vi "verify parameters in a list.vi"(8 "error in (no error)":errorcluster, 11 "Simulated_CCD_Camera in":refnum<class "Sim_Ixon_Ultra.lvclass">) -> (0 "error out":errorcluster, 3 "Simulated_CCD_Camera out":refnum<class "Sim_Ixon_Ultra.lvclass">)   [LabVIEW 2018, in "Sim_Ixon_Ultra.lvclass"]
doc: "Verify if the parameters of the camera are in range\n\nThe operating parameters of the CCDs must be within a predefined range. This function verifies if the values provided for these parameters meet this specification. If not, ACS will not allow to start an exposure."
uses:
  Sim_Ixon_Ultra.lvclass
  C:/Users/Denis/Desktop/S4ACS/S4ACS/Simulated_CCD_Camera/Simulated Camera.lvclass
  Simulated_CCD_Camera/Simulated Camera.lvclass
panel:
  out "New CCD Config":T1
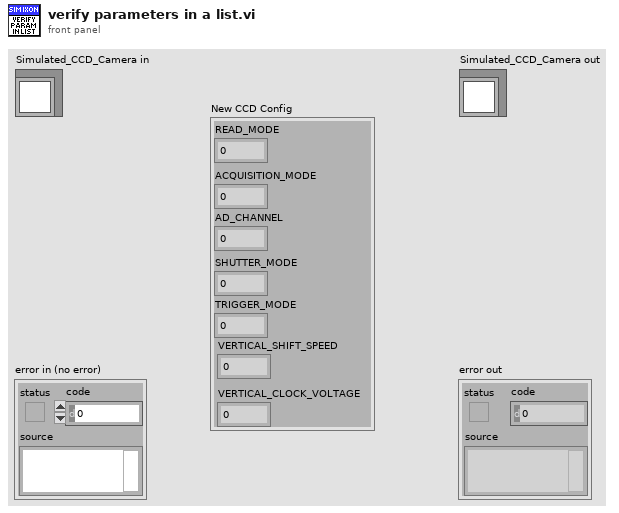
[diagram p1: front panel]
types:
  T1 = cluster{"READ_MODE":u16, "ACQUISITION_MODE":u16, "AD_CHANNEL":u16, "SHUTTER_MODE":u16, "TRIGGER_MODE":u16, "VERTICAL_SHIFT_SPEED":u16, "VERTICAL_CLOCK_VOLTAGE":u16}
  T2 = cluster{"PREAMP":u16, "READOUT_RATE":u16, "VERTICAL_SHIFT_SPEED":u16, "READ_MODE":u16, "VERTICAL_CLOCK_VOLTAGE":u16, "ACQUISITION_MODE":u16, "AD_CHANNEL":u16, "SHUTTER_TTL":u16, "SHUTTER_OPENING_TIME":u16, "SHUTTER_CLOSING_TIME":u16, "SHUTTER_MODE":u16, "TRIGGER_MODE":u16, "VBIN":u16, "INITIAL_LINE":u16, "INITIAL_COLUMN":u16, "FINAL_LINE":u16, "FINAL_COLUMN":u16, "HBIN":u16, "TEMP":u16, "COOLER_POWER_STATUS":u16}
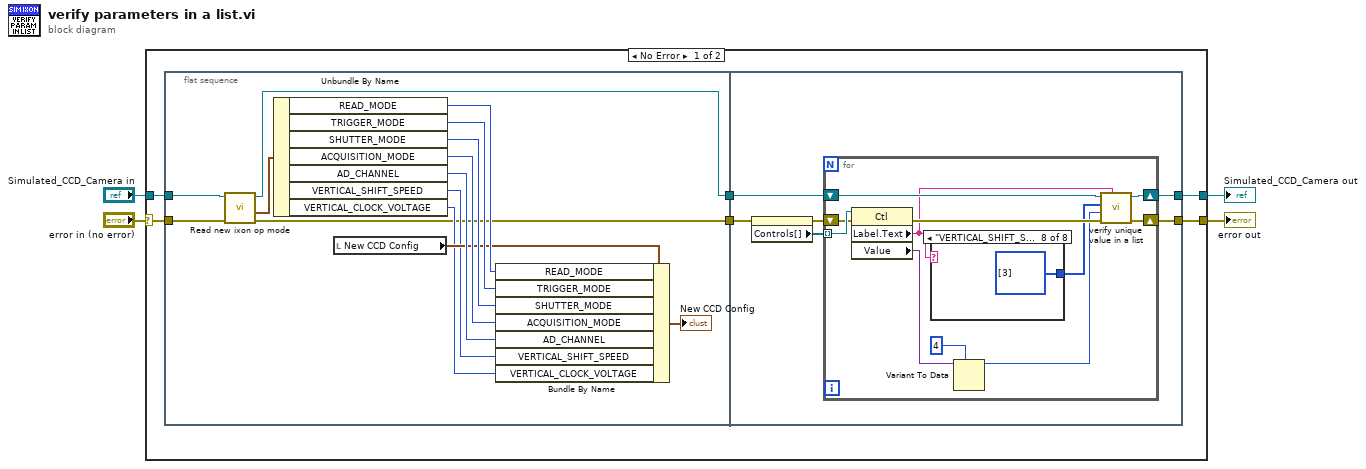
[diagram p0: block diagram]
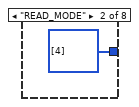
[diagram p3: hidden frame]
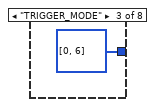
[diagram p4: hidden frame]
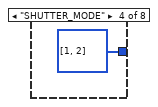
[diagram p5: hidden frame]
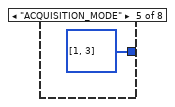
[diagram p6: hidden frame]
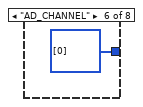
[diagram p7: hidden frame]
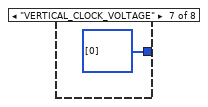
[diagram p8: hidden frame]
diagram:
  n1 = case shown="No Error" "error in (no error)" {
    selector: "error in (no error)" -> [w8 w49]
    tunnel: "Simulated_CCD_Camera in" -> [w7 w50]
    tunnel: [w6 w50] -> w2
    tunnel: [w5 w49] -> w1
    frame No Error {
      n2 = flat-sequence {
        tunnel: w8 -> [w13]
        tunnel: w7 -> [w14]
        tunnel: [w11] -> w10
        tunnel: [w12] -> w9
        tunnel: [w29] -> w5
        tunnel: [w28] -> w6
        tunnel: w10 -> [w30]
        tunnel: w9 -> [w26]
        frame #0 {
          n3 = call-dynamic "Read new ixon op mode.vi"("error in (no error)"=w13, "Sim_Ixon_Ultra in"=w14) -> ("error out"=w12:errorcluster, "new operation mode"=w15:T2, "Sim_Ixon_Ultra out"=w11:refnum<class "Sim_Ixon_Ultra.lvclass">)  [unwired: 6 in, 1 out]
          n4 = Unbundle By Name(w15) -> ("READ_MODE"=w24:u16, "TRIGGER_MODE"=w23:u16, "SHUTTER_MODE"=w22:u16, "ACQUISITION_MODE"=w21:u16, "AD_CHANNEL"=w20:u16, "VERTICAL_SHIFT_SPEED"=w17:u16, "VERTICAL_CLOCK_VOLTAGE"=w16:u16)
          n5 = local read "New CCD Config"() -> (w18:T1)
          n6 = Bundle By Name(cluster=w18, "READ_MODE"=w24, "TRIGGER_MODE"=w23, "SHUTTER_MODE"=w22, "ACQUISITION_MODE"=w21, "AD_CHANNEL"=w20, "VERTICAL_SHIFT_SPEED"=w17, "VERTICAL_CLOCK_VOLTAGE"=w16) -> (→"New CCD Config":T1)
        }
        frame #1 {
          n7 = property on="New CCD Config" class="Clust (strict)"(error in=w26) -> (error out=w25:errorcluster, "Controls[]"=w27:refnum<vi>[])  [unwired: 1 in, 1 out]
          n8 = for {
            shift-right: [w40] -> w29
            shift-left: w25 -> [w37]
            shift-right: [w39] -> w28
            shift-left: w30 -> [w41]
            tunnel: w27 -> [w38] mode=indexing
            n9 = property class="Ctl"(reference=w38, error in=w37) -> (error out=w36:errorcluster, "Label.Text"=w34:string, "Value"=w33:variant)  [unwired: 1 out]
            n10 = case shown="\"VERTICAL_SHIFT_SPEED\"" w34 {
              tunnel: [_ i32[] [4] i32[] [0, 6] i32[] [1, 2] i32[] [1, 3] i32[] [0] i32[] [0] i32[] [3]] -> w35
              frame "False", Default {
              }
              frame "READ_MODE" {
              }
              frame "TRIGGER_MODE" {
              }
              frame "SHUTTER_MODE" {
              }
              frame "ACQUISITION_MODE" {
              }
              frame "AD_CHANNEL" {
              }
              frame "VERTICAL_CLOCK_VOLTAGE" {
              }
              frame "VERTICAL_SHIFT_SPEED" {
              }
            }
            n11 = Variant To Data(type=4, Variant=w33) -> (data=w31:i32)  [unwired: 1 in, 1 out]
            n12 = call "verify unique value in a list.vi"("parameter name"=w34, "error in (no error)"=w36, "value"=w31, "list of values"=w35, "Simulated_CCD_Camera in"=w41) -> ("error out"=w40:errorcluster, "Simulated_CCD_Camera out"=w39:refnum<class "Sim_Ixon_Ultra.lvclass">)  [unwired: 5 in]
          }
        }
      }
    }
    frame Error {
    }
  }
  "error out" <- w1
  "Simulated_CCD_Camera out" <- w2
